vi "Calculate COB-ID from EBNF.vi"(8 "error in":errorcluster, 10 "Node ID":u8, 11 "ENBF":string) -> (0 "error out":errorcluster, 3 "COB-ID":u32)   [LabVIEW 2020, in "CANopen.lvlib" / "PDO Communication Parameter.lvclass"]
doc: "Parses Node-ID from Extended Backus-Naur formula in PDO communication sub-index 1 defaultvalue"
uses:
  PDO Communication Parameter.lvclass
  PDO Communication Parameter.lvclass/PDO Communication Parameter.ctl
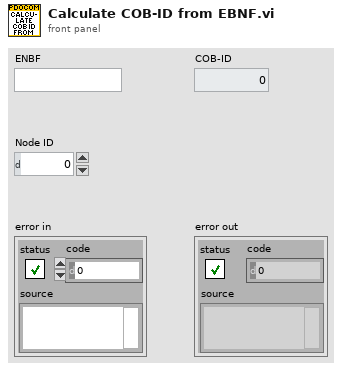
[diagram p1: front panel]
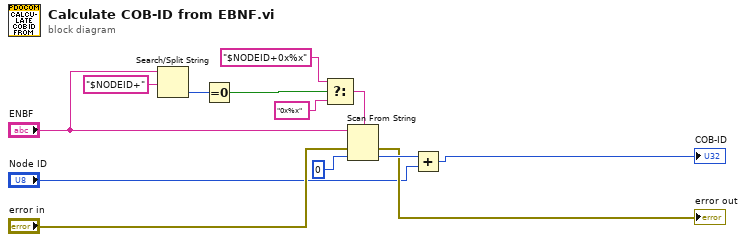
[diagram p0: block diagram]
diagram:
  n1 = Search/Split String(string="ENBF", search string/char (-)="$NODEID+") -> (offset of match=w5:i32)  [unwired: 1 in, 2 out]
  n2 = Equal To 0?(x=w5) -> (x = 0?=w4:bool)
  n3 = Select(t="$NODEID+0x%x" ("format string"), s=w4, f="0x%x" ("format string")) -> (s? t:f=w6:string)
  n4 = Scan From String(format string=w6, input string="ENBF", error in="error in", default 1=u32 0) -> (error out=→"error out":errorcluster, output 1=w11:u32)  [unwired: 1 in, 2 out]
  n5 = Add(x=w11, y="Node ID") -> (x+y=→"COB-ID":u32)
